vi "SUB_Write_GEN4_Init_data_V2_0_1 - A1.vi"(5 "Interval Time":enum16{"10ms", "33ms", "50ms"}(ring), 7 "Mode":T9, 11 "Port-act 1":refnum<visa-resource-name>="COM8") -> (0 "원소":u8, 1 "불리언 2":bool)   [LabVIEW 2015]
uses:
  Lib_Bled112 toolkit/ble_functions/ble_write_by_handle_uint8array.vi
  Lib_Bled112 toolkit/type_def/address_type.ctl
  Lib_Bled112 toolkit/type_def/connection_status_bundle.ctl
  Cluster Type/Device information.ctl
  Cluster Type/Cal information.ctl
  Cluster Type/PCAP zero information.ctl
  Type definition/write_mode.ctl
  Cluster Type/add data1.ctl
  Cluster Type/add data2.ctl
  Cluster Type/add data3.ctl
  Cluster Type/add data4.ctl
  Cluster Type/Acclerometer value(0, 45).ctl
  Cluster Type/Acclerometer value(90, 180).ctl
panel:
  in  "불리언":bool
  in  "Acclerometer value(90, 180)":T1 {"Check sum" format="%x"; "Reserved_2" format="%x"; "Reserved_1" format="%x"; "second counter_2" format="%x"; "Acc. Z_90 val_L" format="%x"; "second counter_1" format="%x"; "Acc. Z_180 val_L" format="%x"; "Acc. Z_180 val_H" format="%x"; "Acc. Y_180 val_L" format="%x"; "Acc. Y_180 val_H" format="%x"; "Acc. X_180 val_L" format="%x"; "Acc. X_180 val_H" format="%x"; "Acc. Z_90 val_H" format="%x"; "Acc. Y_90 val_L" format="%x"; "Acc. Y_90 val_H" format="%x"; "Acc. X_90 val_L" format="%x"; "Acc. X_90 val_H" format="%x"; "Packet ID" format="%x"}
  in  "Acclerometer value(0, 45)":T2 {"Check sum" format="%x"; "Reserved_4" format="%x"; "Reserved_3" format="%x"; "Reserved_2" format="%x"; "Acc. Z_0 val_L" format="%x"; "Reserved_1" format="%x"; "Acc. Z_45 val_L" format="%x"; "Acc. Z_45 val_H" format="%x"; "Acc. Y_45 val_L" format="%x"; "Acc. Y_45 val_H" format="%x"; "Acc. X_45 val_L" format="%x"; "Acc. X_45 val_H" format="%x"; "Acc. Z_0 val_H" format="%x"; "Acc. Y_0 val_L" format="%x"; "Acc. Y_0 val_H" format="%x"; "Acc. X_0 val_L" format="%x"; "Acc. X_0 val_H" format="%x"; "Packet ID" format="%x"}
  in  "data4":T3 {"Check sum" format="%x"; "Reserved_8" format="%x"; "Reserved_7" format="%x"; "Reserved_6" format="%x"; "Cal_Compart. B_16_2" format="%x"; "Reserved_5" format="%x"; "Reserved_4" format="%x"; "Reserved_3" format="%x"; "Reserved_2" format="%x"; "Reserved_1" format="%x"; "Cal_Compart. B_16_4" format="%x"; "Cal_Compart. B_16_3" format="%x"; "Cal_Compart. B_16_1" format="%x"; "Cal_Compart. A_16_4" format="%x"; "Cal_Compart. A_16_3" format="%x"; "Cal_Compart. A_16_2" format="%x"; "Cal_Compart. A_16_1" format="%x"; "Packet ID" format="%x"}
  in  "data3":T4 {"Check sum" format="%x"; "Cal_Compart. B_14_4" format="%x"; "Cal_Compart. B_14_3" format="%x"; "Cal_Compart. B_14_2" format="%x"; "Cal_Compart. B_13_2" format="%x"; "Cal_Compart. B_14_1" format="%x"; "Cal_Compart. A_14_4" format="%x"; "Cal_Compart. A_14_3" format="%x"; "Cal_Compart. A_14_2" format="%x"; "Cal_Compart. A_14_1" format="%x"; "Cal_Compart. B_13_4" format="%x"; "Cal_Compart. B_13_3" format="%x"; "Cal_Compart. B_13_1" format="%x"; "Cal_Compart. A_13_4" format="%x"; "Cal_Compart. A_13_3" format="%x"; "Cal_Compart. A_13_2" format="%x"; "Cal_Compart. A_13_1" format="%x"; "Packet ID" format="%x"}
  in  "data2":T5 {"Check sum" format="%x"; "Cal_Compart. B_12_4" format="%x"; "Cal_Compart. B_12_3" format="%x"; "Cal_Compart. B_12_2" format="%x"; "Cal_Compart. B_11_2" format="%x"; "Cal_Compart. B_12_1" format="%x"; "Cal_Compart. A_12_4" format="%x"; "Cal_Compart. A_12_3" format="%x"; "Cal_Compart. A_12_2" format="%x"; "Cal_Compart. A_12_1" format="%x"; "Cal_Compart. B_11_4" format="%x"; "Cal_Compart. B_11_3" format="%x"; "Cal_Compart. B_11_1" format="%x"; "Cal_Compart. A_11_4" format="%x"; "Cal_Compart. A_11_3" format="%x"; "Cal_Compart. A_11_2" format="%x"; "Cal_Compart. A_11_1" format="%x"; "Packet ID" format="%x"}
  in  "data1":T6 {"Check sum" format="%x"; "Reserved_6" format="%x"; "Reserved_5" format="%x"; "Reserved_4" format="%x"; "Cal_Compart. A_10_4" format="%x"; "Reserved_3" format="%x"; "Reserved_2" format="%x"; "Reserved_1" format="%x"; "Cal_Compart. B_10_4" format="%x"; "Cal_Compart. B_10_3" format="%x"; "Cal_Compart. B_10_2" format="%x"; "Cal_Compart. B_10_1" format="%x"; "Cal_Compart. A_10_3" format="%x"; "Cal_Compart. A_10_2" format="%x"; "Cal_Compart. A_10_1" format="%x"; "Operative Side" format="%x"; "Firmware Revision" format="%x"; "Packet ID" format="%x"}
  in  "Delay(ms)":u32=3
  in  "Connection Status":T7={"MAC Address"="F8:B8:54:EF:76:8D", "cnx handle"=0, "cnx flags"=5, "Address Type"=1, "Connection Interval (ms)"=8, "Timeout(ms)"=1000, "Latency"=0, "bonding handle"=255} {"Address Type" items=["Public", "Random"]}
  in  "PCAP zero information":T10 {"Check sum" format="%x"; "Sensor 8_L" format="%x"; "Sensor 8_H" format="%x"; "Sensor 7_L" format="%x"; "Sensor 7_H" format="%x"; "Sensor 6_L" format="%x"; "Sensor 6_H" format="%x"; "Sensor 5_L" format="%x"; "Sensor 5_H" format="%x"; "Sensor 4_L" format="%x"; "Sensor 4_H" format="%x"; "Sensor 3_L" format="%x"; "Sensor 3_H" format="%x"; "Sensor 2_L" format="%x"; "Sensor 2_H" format="%x"; "Sensor 1_L" format="%x"; "Sensor 1_H" format="%x"; "Packet ID" format="%x"}
  in  "Cal information":T11 {"Check sum" format="%x"; "Voltage L 2.8V" format="%x"; "Voltage H 2.8V" format="%x"; "Voltage L 3.1V" format="%x"; "Acc Z_L_Cal" format="%x"; "Voltage H 3.1V" format="%x"; "Gyro Z_L_Cal" format="%x"; "Gyro Z_H_Cal" format="%x"; "Gyro Y_L_Cal" format="%x"; "Gyro Y_H_Cal" format="%x"; "Gyro X_L_Cal" format="%x"; "Gyro X_H_Cal" format="%x"; "Acc Z_H_Cal" format="%x"; "Acc Y_L_Cal" format="%x"; "Acc Y_H_Cal" format="%x"; "Acc X_L_Cal" format="%x"; "Acc X_H_Cal" format="%x"; "Packet ID" format="%x"}
  in  "Device information":T12 {"Check sum 2" format="%x"; "Device Type L" format="%x"; "Device Type H" format="%x"; "Check sum" format="%x"; "Scale B" format="%x"; "Scale A" format="%x"; "Manufacturer Lot ID 4" format="%x"; "Manufacturer Lot ID 3" format="%x"; "Manufacturer Lot ID 2" format="%x"; "Manufacturer Lot ID 1" format="%x"; "Day" format="%x"; "Month" format="%x"; "Year" format="%x"; "Device ID 4" format="%x"; "Device ID 3" format="%x"; "Device ID 2" format="%x"; "Device ID 1" format="%x"; "Packet ID" format="%x"}
  # "(Device Type is divided 1byte)"
  # "=> Sensor Offset Valure"
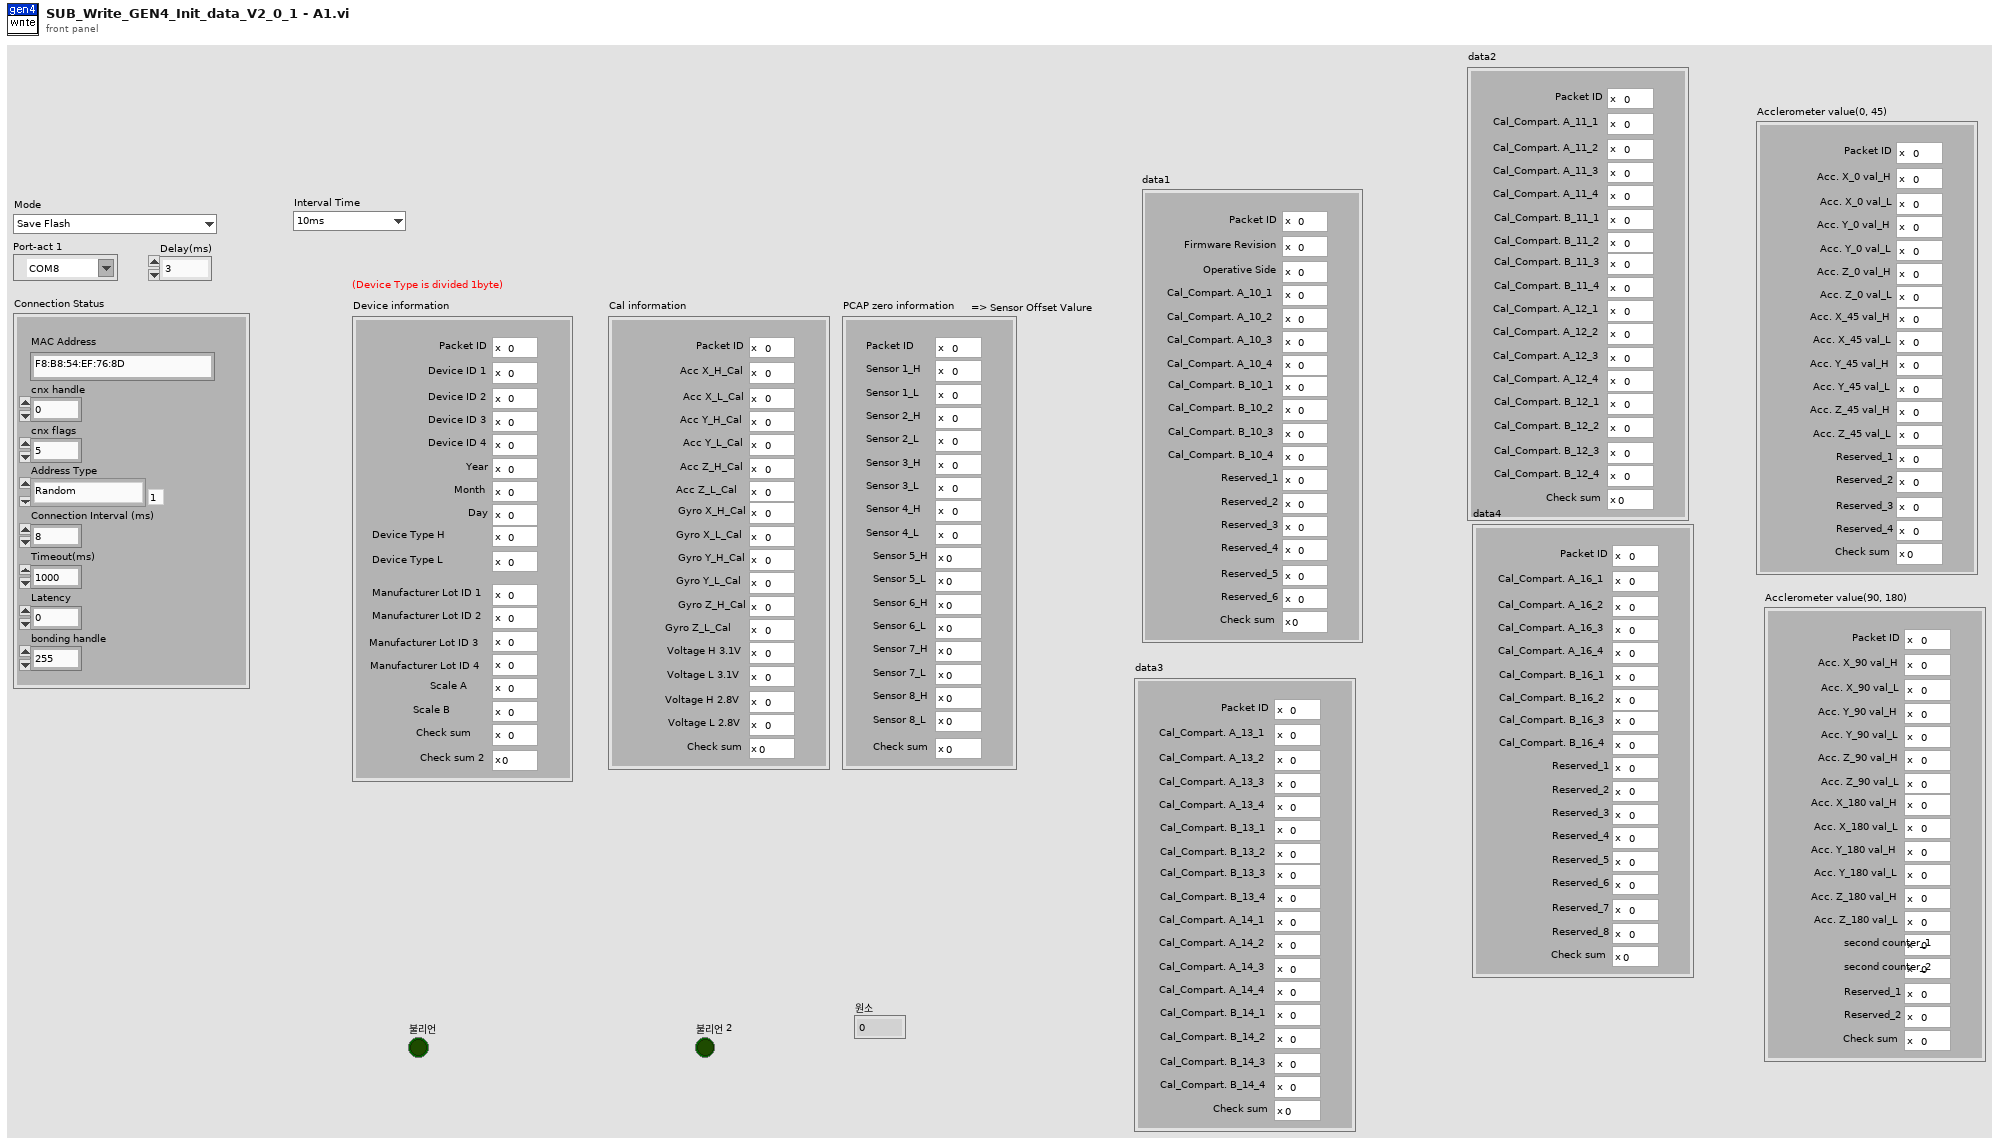
[diagram p1: front panel]
types:
  T1 = typedef "Acclerometer value(90, 180).ctl" = cluster{"Packet ID":u8, "Acc. X_90 val_H":u8, "Acc. X_90 val_L":u8, "Acc. Y_90 val_H":u8, "Acc. Y_90 val_L":u8, "Acc. Z_90 val_H":u8, "Acc. Z_90 val_L":u8, "Acc. X_180 val_H":u8, "Acc. X_180 val_L":u8, "Acc. Y_180 val_H":u8, "Acc. Y_180 val_L":u8, "Acc. Z_180 val_H":u8, "Acc. Z_180 val_L":u8, "second counter_1":u8, "second counter_2":u8, "Reserved_1":u8, "Reserved_2":u8, "Check sum":u8}
  T2 = typedef "Acclerometer value(0, 45).ctl" = cluster{"Packet ID":u8, "Acc. X_0 val_H":u8, "Acc. X_0 val_L":u8, "Acc. Y_0 val_H":u8, "Acc. Y_0 val_L":u8, "Acc. Z_0 val_H":u8, "Acc. Z_0 val_L":u8, "Acc. X_45 val_H":u8, "Acc. X_45 val_L":u8, "Acc. Y_45 val_H":u8, "Acc. Y_45 val_L":u8, "Acc. Z_45 val_H":u8, "Acc. Z_45 val_L":u8, "Reserved_1":u8, "Reserved_2":u8, "Reserved_3":u8, "Reserved_4":u8, "Check sum":u8}
  T3 = typedef "add data4.ctl" = cluster{"Packet ID":u8, "Cal_Compart. A_16_1":u8, "Cal_Compart. A_16_2":u8, "Cal_Compart. A_16_3":u8, "Cal_Compart. A_16_4":u8, "Cal_Compart. B_16_1":u8, "Cal_Compart. B_16_2":u8, "Cal_Compart. B_16_3":u8, "Cal_Compart. B_16_4":u8, "Reserved_1":u8, "Reserved_2":u8, "Reserved_3":u8, "Reserved_4":u8, "Reserved_5":u8, "Reserved_6":u8, "Reserved_7":u8, "Reserved_8":u8, "Check sum":u8}
  T4 = typedef "add data3.ctl" = cluster{"Packet ID":u8, "Cal_Compart. A_13_1":u8, "Cal_Compart. A_13_2":u8, "Cal_Compart. A_13_3":u8, "Cal_Compart. A_13_4":u8, "Cal_Compart. B_13_1":u8, "Cal_Compart. B_13_2":u8, "Cal_Compart. B_13_3":u8, "Cal_Compart. B_13_4":u8, "Cal_Compart. A_14_1":u8, "Cal_Compart. A_14_2":u8, "Cal_Compart. A_14_3":u8, "Cal_Compart. A_14_4":u8, "Cal_Compart. B_14_1":u8, "Cal_Compart. B_14_2":u8, "Cal_Compart. B_14_3":u8, "Cal_Compart. B_14_4":u8, "Check sum":u8}
  T5 = typedef "add data2.ctl" = cluster{"Packet ID":u8, "Cal_Compart. A_11_1":u8, "Cal_Compart. A_11_2":u8, "Cal_Compart. A_11_3":u8, "Cal_Compart. A_11_4":u8, "Cal_Compart. B_11_1":u8, "Cal_Compart. B_11_2":u8, "Cal_Compart. B_11_3":u8, "Cal_Compart. B_11_4":u8, "Cal_Compart. A_12_1":u8, "Cal_Compart. A_12_2":u8, "Cal_Compart. A_12_3":u8, "Cal_Compart. A_12_4":u8, "Cal_Compart. B_12_1":u8, "Cal_Compart. B_12_2":u8, "Cal_Compart. B_12_3":u8, "Cal_Compart. B_12_4":u8, "Check sum":u8}
  T6 = typedef "add data1.ctl" = cluster{"Packet ID":u8, "Firmware Revision":u8, "Operative Side":u8, "Cal_Compart. A_10_1":u8, "Cal_Compart. A_10_2":u8, "Cal_Compart. A_10_3":u8, "Cal_Compart. A_10_4":u8, "Cal_Compart. B_10_1":u8, "Cal_Compart. B_10_2":u8, "Cal_Compart. B_10_3":u8, "Cal_Compart. B_10_4":u8, "Reserved_1":u8, "Reserved_2":u8, "Reserved_3":u8, "Reserved_4":u8, "Reserved_5":u8, "Reserved_6":u8, "Check sum":u8}
  T7 = typedef "connection_status_bundle.ctl" = cluster{"MAC Address":string, "cnx handle":u8, "cnx flags":u8, "Address Type":T8, "Connection Interval (ms)":u16, "Timeout(ms)":u16, "Latency":u16, "bonding handle":u8}
  T8 = typedef "address_type.ctl" = u8
  T9 = typedef "write_mode.ctl" = enum16{"Save Flash", "Visa save", "Interval Change"}
  T10 = typedef "PCAP zero information.ctl" = cluster{"Packet ID":u8, "Sensor 1_H":u8, "Sensor 1_L":u8, "Sensor 2_H":u8, "Sensor 2_L ":u8, "Sensor 3_H":u8, "Sensor 3_L":u8, "Sensor 4_H":u8, "Sensor 4_L":u8, "Sensor 5_H":u8, "Sensor 5_L":u8, "Sensor 6_H":u8, "Sensor 6_L":u8, "Sensor 7_H":u8, "Sensor 7_L":u8, "Sensor 8_H":u8, "Sensor 8_L":u8, "Check sum":u8}
  T11 = typedef "Cal information.ctl" = cluster{"Packet ID":u8, "Acc X_H_Cal":u8, "Acc X_L_Cal":u8, "Acc Y_H_Cal":u8, "Acc Y_L_Cal":u8, "Acc Z_H_Cal":u8, "Acc Z_L_Cal":u8, "Gyro X_H_Cal":u8, "Gyro X_L_Cal":u8, "Gyro Y_H_Cal":u8, "Gyro Y_L_Cal":u8, "Gyro Z_H_Cal":u8, "Gyro Z_L_Cal":u8, "Voltage H 3.1V":u8, "Voltage L 3.1V":u8, "Voltage H 2.8V":u8, "Voltage L 2.8V":u8, "Check sum":u8}
  T12 = typedef "Device information.ctl" = cluster{"Packet ID":u8, "Device ID 1":u8, "Device ID 2":u8, "Device ID 3":u8, "Device ID 4":u8, "Year":u8, "Month":u8, "Day":u8, "Device Type H":u8, "Device Type L":u8, "Manufacturer Lot ID 1":u8, "Manufacturer Lot ID 2":u8, "Manufacturer Lot ID 3":u8, "Manufacturer Lot ID 4":u8, "Scale A":u8, "Scale B":u8, "Check sum":u8, "Check sum 2":u8}
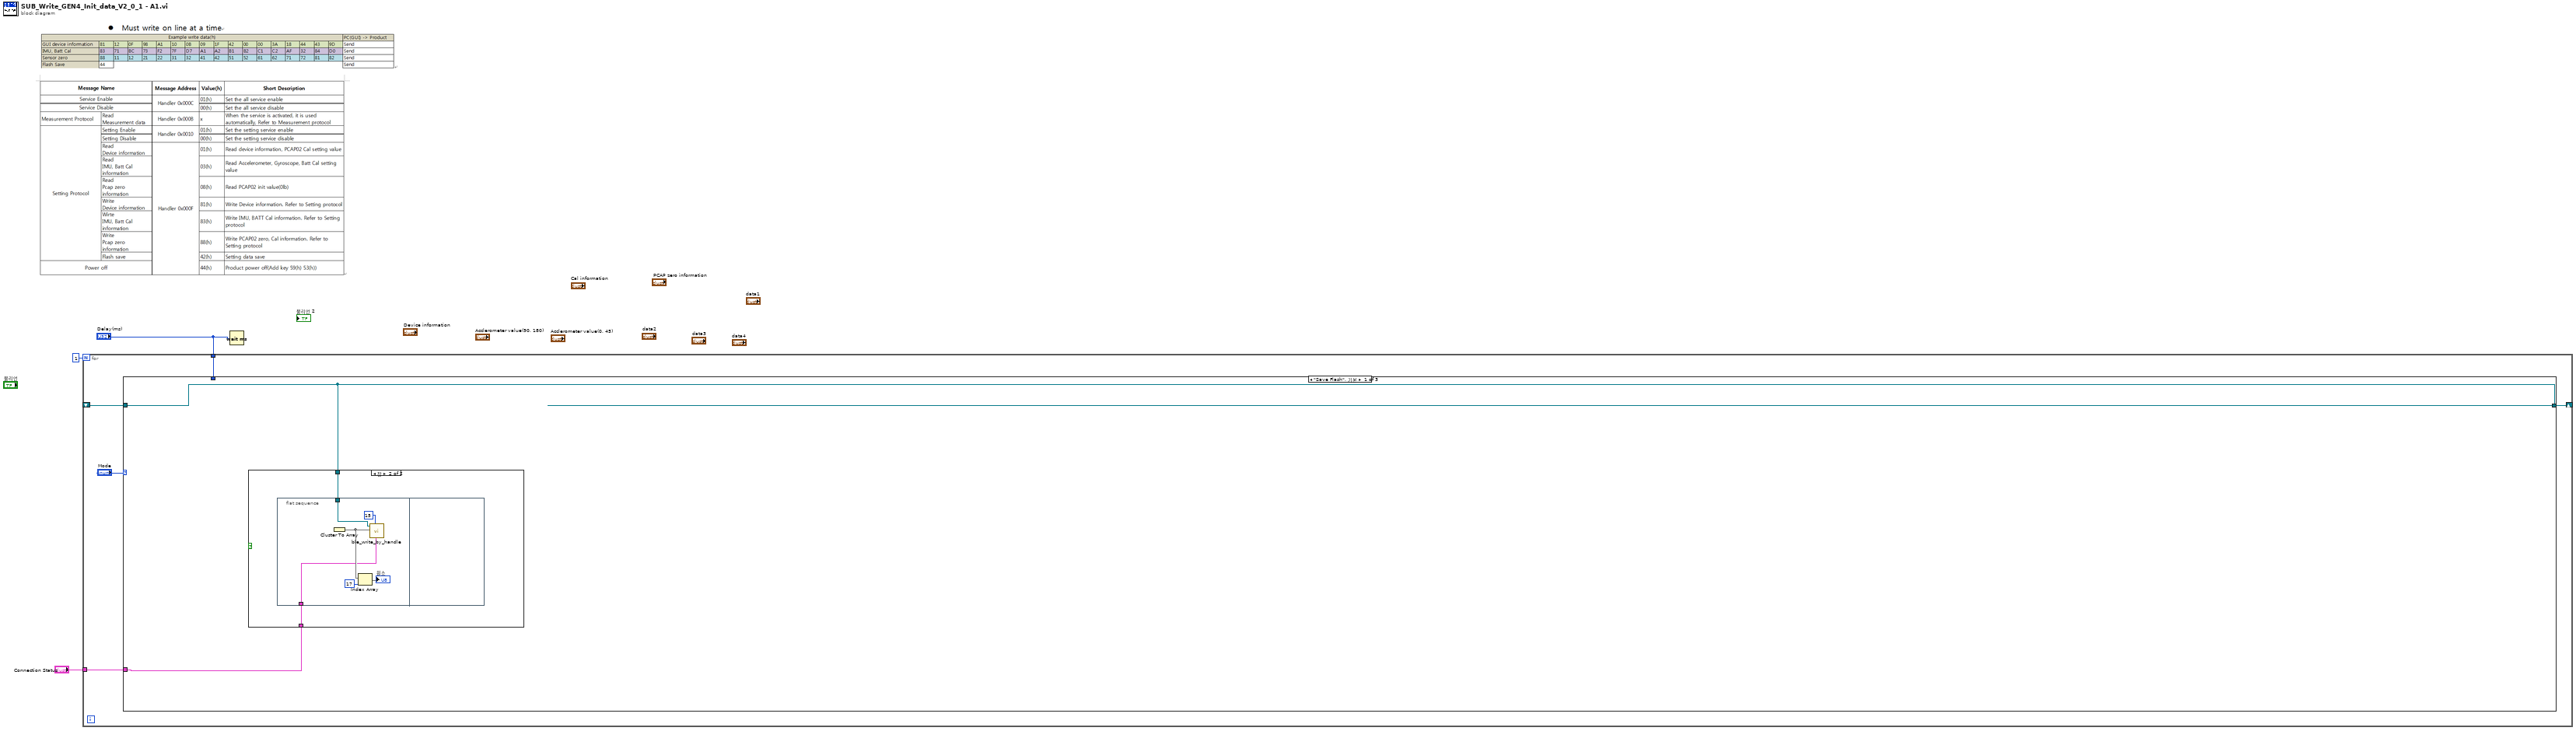
[diagram p0: block diagram]
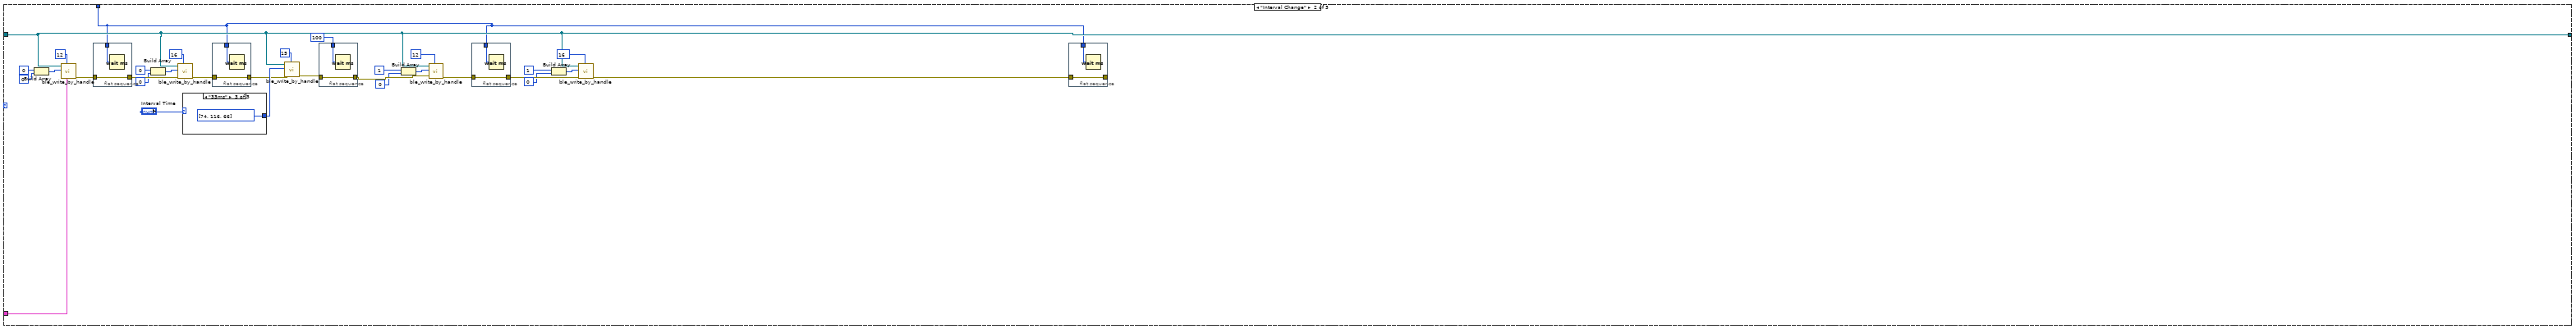
[diagram p3: hidden frame]
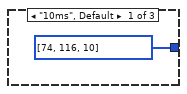
[diagram p4: hidden frame]
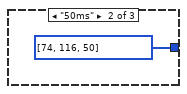
[diagram p5: hidden frame]
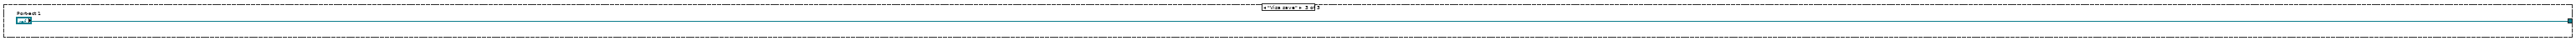
[diagram p6: hidden frame]
diagram:
  n1 = for {
    N: 1 -> [_]
    shift-right: [w8] -> _
    shift-left: _ -> [w7]
    tunnel: "Connection Status" -> [w6]
    tunnel: "Delay(ms)" -> [w5]
    n2 = case shown="\"Save Flash\", 기본" "Mode" {
      tunnel: [w11 w37 "Port-act 1"] -> w8
      tunnel: w7 -> [w11 w37 _]
      tunnel: w6 -> [w10 w50 _]
      tunnel: w5 -> [_ w25 _]
      frame "Save Flash", Default {
        n3 = case shown="참" {
          selector: _ -> [_ _]
          tunnel: w11 -> [_ w13]
          tunnel: w10 -> [_ w12]
          frame False {
          }
          frame True {
            n4 = flat-sequence {
              tunnel: w13 -> [w15]
              tunnel: w12 -> [w14]
              frame #0 {
                n5 = Cluster To Array() -> (array=w16:void[])  [unwired: 1 in]
                n6 = Index Array(array=w16, index=17 ("인덱스")) -> (element=→"원소")
                n7 = call-poly "ble_write_by_handle.vi"("Connection Status"=w14, "Handle"=u16 15, "data (uint8array)"=w16, "COM Bluegiga in"=w15) -> ()  [unwired: 6 in, 2 out]
              }
              frame #1 {
              }
            }
          }
        }
      }
      frame "Interval Change" {
        n8 = Build Array(u16 0 ("Handle"), u16 0 ("Handle")) -> (w48:u16[])
        n9 = call-poly "ble_write_by_handle.vi"("Connection Status"=w50, "Handle"=u16 12, "data (uint8array)"=w48, "COM Bluegiga in"=w37) -> ("error out"=w33:errorcluster)  [unwired: 6 in, 1 out]
        n10 = flat-sequence {
          tunnel: w25 -> [w61]
          tunnel: [w60] -> w34
          tunnel: w33 -> [w60]
          frame #0 {
            n11 = Wait (ms)(milliseconds to wait=w61) -> ()  [unwired: 1 out]
          }
        }
        n12 = Build Array(u16 0 ("Handle"), u16 0 ("Handle")) -> (w47:u16[])
        n13 = call-poly "ble_write_by_handle.vi"("Handle"=u16 16, "error in (no error)"=w34, "data (uint8array)"=w47, "COM Bluegiga in"=w37) -> ("error out"=w32:errorcluster)  [unwired: 6 in, 1 out]
        n14 = case shown="\"33ms\"" "Interval Time" {
          tunnel: [u8[] [74, 116, 10] u8[] [74, 116, 50] u8[] [74, 116, 66]] -> w35
          frame "10ms", Default {
          }
          frame "50ms" {
          }
          frame "33ms" {
          }
        }
        n15 = flat-sequence {
          tunnel: w25 -> [w59]
          tunnel: [w58] -> w31
          tunnel: w32 -> [w58]
          frame #0 {
            n16 = Wait (ms)(milliseconds to wait=w59) -> ()  [unwired: 1 out]
          }
        }
        n17 = call-poly "ble_write_by_handle.vi"("Handle"=u16 15, "error in (no error)"=w31, "data (uint8array)"=w35, "COM Bluegiga in"=w37) -> ("error out"=w30:errorcluster)  [unwired: 6 in, 1 out]
        n18 = flat-sequence {
          tunnel: u32 100 ("대기 시간(ms)") -> [w57]
          tunnel: [w56] -> w29
          tunnel: w30 -> [w56]
          frame #0 {
            n19 = Wait (ms)(milliseconds to wait=w57) -> ()  [unwired: 1 out]
          }
        }
        n20 = Build Array(u16 1 ("Handle"), u16 0 ("Handle")) -> (w41:u16[])
        n21 = call-poly "ble_write_by_handle.vi"("Handle"=u16 12, "error in (no error)"=w29, "data (uint8array)"=w41, "COM Bluegiga in"=w37) -> ("error out"=w28:errorcluster)  [unwired: 6 in, 1 out]
        n22 = flat-sequence {
          tunnel: w25 -> [w55]
          tunnel: [w54] -> w27
          tunnel: w28 -> [w54]
          frame #0 {
            n23 = Wait (ms)(milliseconds to wait=w55) -> ()  [unwired: 1 out]
          }
        }
        n24 = Build Array(u16 1 ("Handle"), u16 0 ("Handle")) -> (w42:u16[])
        n25 = call-poly "ble_write_by_handle.vi"("Handle"=u16 16, "error in (no error)"=w27, "data (uint8array)"=w42, "COM Bluegiga in"=w37) -> ("error out"=w26:errorcluster)  [unwired: 6 in, 1 out]
        n26 = flat-sequence {
          tunnel: w25 -> [w53]
          tunnel: [w52] -> _
          tunnel: w26 -> [w52]
          frame #0 {
            n27 = Wait (ms)(milliseconds to wait=w53) -> ()  [unwired: 1 out]
          }
        }
      }
      frame "Visa save" {
      }
    }
  }
  n28 = Wait (ms)(milliseconds to wait="Delay(ms)") -> ()  [unwired: 1 out]
